vi "purficateur de liquides.vi"(1 "Nb de litres recus":i32) -> (0 "nb de litres purifies":dbl)   [LabVIEW 2020]
panel:
  out "x-y":dbl
  out "pH":dbl
  out "acide":bool
  out "neutre":bool
  out "basique":bool
  in  "Bouton OK 3":bool
  out "Bouton OK 2":bool
  out "Booléen 5":bool
  out "Booléen 4":bool
  out "Booléen 3":bool
  out "Booléen 2":bool
  out "Booléen":bool
  out "Réservoir 2":dbl(slide) scale=0.0..10.0
  out "Bouton OK":bool
  out "Réservoir":dbl(slide) scale=0.0..10.0
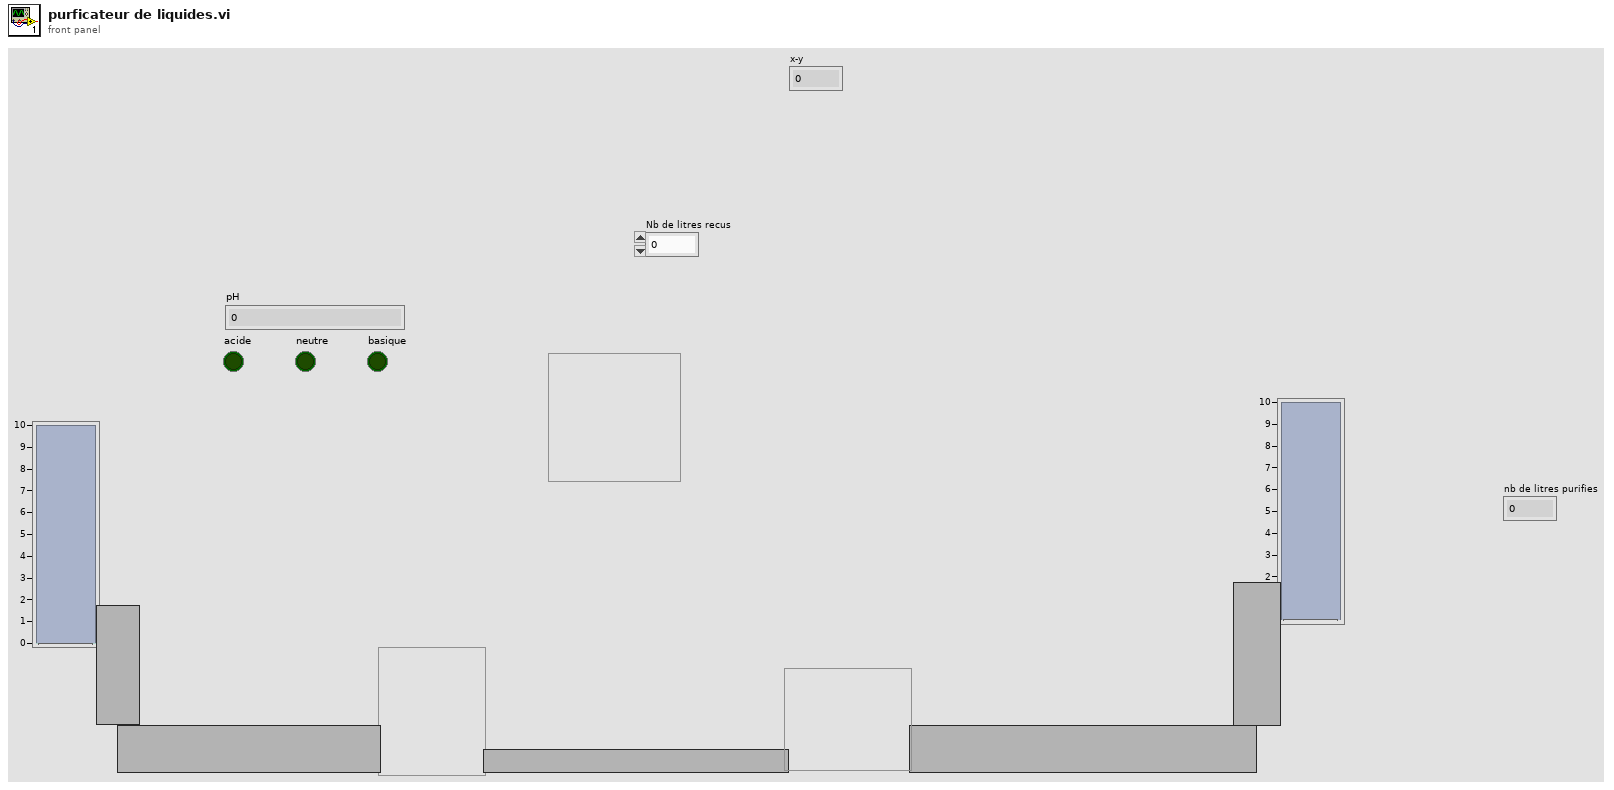
[diagram p1: front panel]
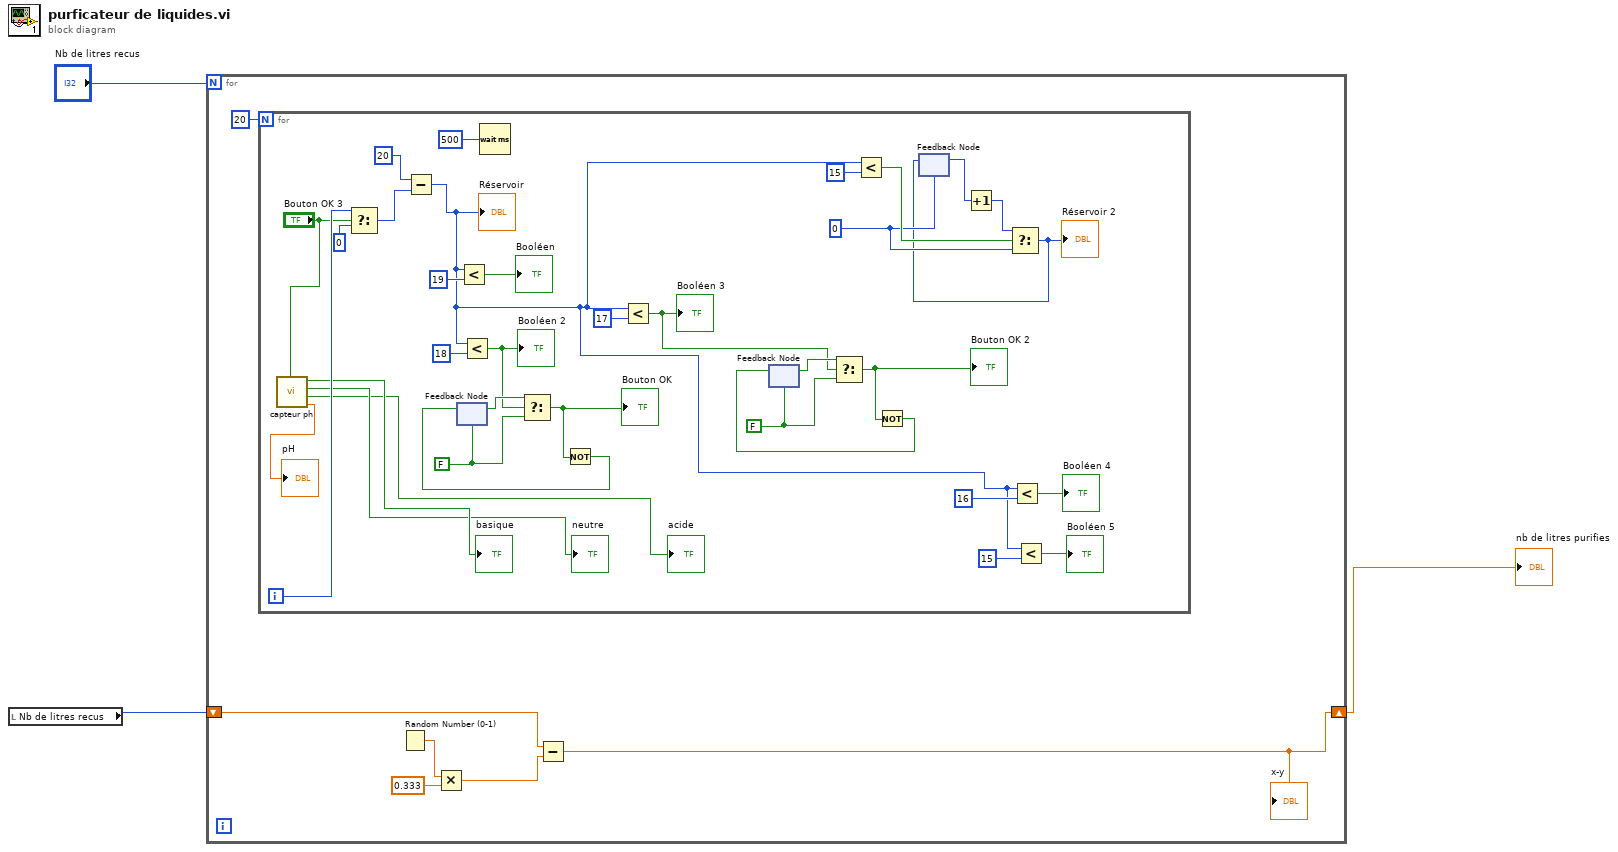
[diagram p0: block diagram]
diagram:
  n1 = local read "Nb de litres recus"() -> (w2:i32)
  n2 = for {
    N: "Nb de litres recus" -> [_]
    shift-right: [w4] -> w1
    shift-left: w2 -> [w6]
    n3 = for {
      N: 20 -> [_]
      i -> [w34]
      w18 = 0 ("y")
      w29 = FALSE
      w37 = FALSE
      n4 = call "capteur ph.vi"("Bouton OK"="Bouton OK 3") -> (">"=→"basique":bool, "="=→"neutre":bool, "<"=→"acide":bool, "Numérique"=→"pH":dbl)
      n5 = Select(t=w34, s="Bouton OK 3", f=0 ("cas faux")) -> (s? t:f=w32:i32)
      n6 = Subtract(x=20, y=w32) -> (x-y=w20:i32)
      "Réservoir" <- w20
      n7 = feedback #1(w37) -> (w39:bool)
      n8 = Less?(x=w20, y=19) -> (x < y?=→"Booléen":bool)
      n9 = Less?(x=w20, y=18) -> (x < y?=w38:bool)
      "Booléen 2" <- w38
      n10 = Wait (ms)(milliseconds to wait=u32 500 ("valeur de l'horloge en ms")) -> ()  [unwired: 1 out]
      n11 = Select(t=w39, s=w38, f=w37) -> (s? t:f=w36:bool)
      "Bouton OK" <- w36
      n12 = Not(x=w36) -> (.not. x?=w35:bool)
      n13 = feedback-in #1(w35) -> ()
      n14 = Less?(x=w20, y=17) -> (x < y?=w27:bool)
      "Booléen 3" <- w27
      n15 = feedback #2(w29) -> (w30:bool)
      n16 = Select(t=w30, s=w27, f=w29) -> (s? t:f=w26:bool)
      "Bouton OK 2" <- w26
      n17 = Less?(x=w20, y=15) -> (x < y?=w19:bool)
      n18 = Not(x=w26) -> (.not. x?=w28:bool)
      n19 = feedback-in #2(w28) -> ()
      n20 = feedback #3(w18) -> (w17:i32)
      n21 = Increment(x=w17) -> (x+1=w16:i32)
      n22 = Select(t=w16, s=w19, f=w18) -> (s? t:f=w15:i32)
      "Réservoir 2" <- w15
      n23 = feedback-in #3(w15) -> ()
      n24 = Less?(x=w20, y=16) -> (x < y?=→"Booléen 4":bool)
      n25 = Less?(x=w20, y=15) -> (x < y?=→"Booléen 5":bool)
    }
    n26 = Random Number (0-1)() -> (number: 0 to 1=w8:dbl)
    n27 = Multiply(x=w8, y=0.333) -> (x*y=w5:dbl)
    n28 = Subtract(x=w6, y=w5) -> (x-y=w4:dbl)
    "x-y" <- w4
  }
  "nb de litres purifies" <- w1
